vi "Get Motor Setpoint Value.vi"(8 "error in (no error)":errorcluster, 10 "state mode":T1 items=["undefined", "angle", "velocity"], 11 "motor communication in":refnum<class "NI_Robotics_Motor Communication Val.lvclass">) -> (0 "error out":errorcluster, 1 "failed?":bool, 2 "value":dbl, 3 "motor communication out":refnum<class "NI_Robotics_Motor Communication Val.lvclass">)   [LabVIEW 2017, in "NI_Robotics_Motor Communication Val.lvclass"]
uses:
  <vilib>/robotics/Actuation/Motor Communication Val/NI_Robotics_Motor Communication Val.lvclass
  <vilib>/robotics/Actuation/Motor Communication/Motor State Mode.ctl
  <vilib>/robotics/Actuation/Motor Communication Val/NI_Robotics_Motor Communication Val.lvclass/NI_Robotics_Motor Communication Val.ctl
  <vilib>/robotics/Actuation/Motor Communication/NI_Robotics_Motor Communication.lvclass
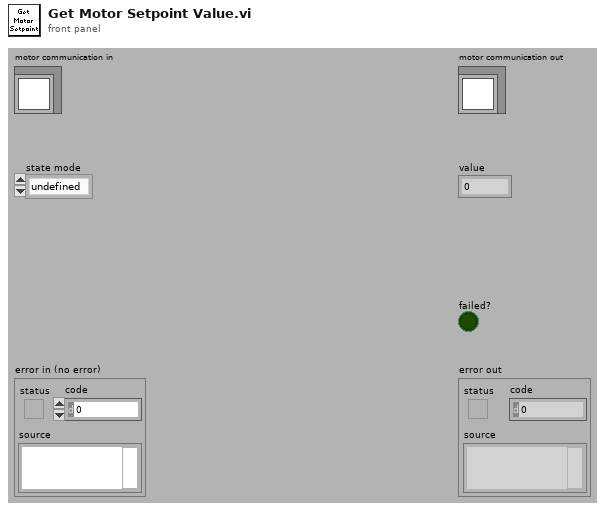
[diagram p1: front panel]
types:
  T1 = typedef "NI_Robotics_Motor Communication.lvclass/Motor State Mode.ctl" = u16
  T2 = typedef "NI_Robotics_Motor Communication.lvclass/Motor State Value.ctl" = cluster{"angle":dbl, "velocity":dbl, "state mode":T1}
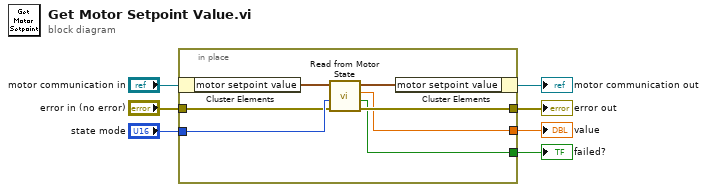
[diagram p0: block diagram]
diagram:
  n1 = in-place {
    in-place-border: "state mode" -> [w12]
    in-place-border: "error in (no error)" -> [w11]
    in-place-border: [w10] -> w4
    in-place-border: [w9] -> w3
    in-place-border: [w8] -> w1
    n2 = in-place-cluster #1("motor communication in") -> ("motor setpoint value"=w14:T2)
    n3 = call <vilib>:"Read from Motor State.vi"("error in (no error)"=w11, "state mode"=w12, "motor state in"=w14) -> ("error out"=w10:errorcluster, "failed?"=w8:bool, "value"=w9:dbl, "motor state out"=w13:T2)  [unwired: 5 in]
    n4 = in-place-cluster #1("motor setpoint value"=w13) -> (→"motor communication out":refnum<class "NI_Robotics_Motor Communication Val.lvclass">)
  }
  "error out" <- w4
  "failed?" <- w1
  "value" <- w3
